vi "Create Ramp Array.vi"(0 "Start":dbl, 5 "Stop":dbl=1.0, 7 "Step":dbl, 11 "Error In":errorcluster) -> (4 "Ramp Pattern":dbl[](array[numeric]), 15 "Error Out":errorcluster)   [LabVIEW 2013]
uses:
  <vilib>/Analysis/1siggen.llb/Ramp Pattern by Delta.vi
  <vilib>/Analysis/NI_AALBase.lvlib
panel:
  out "samples":i32
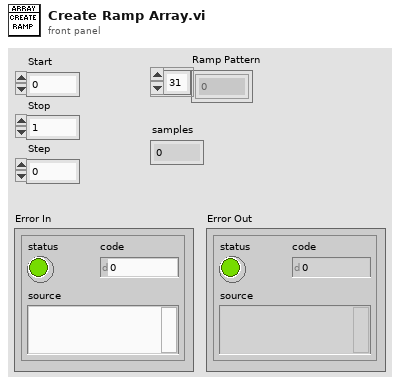
[diagram p1: front panel]
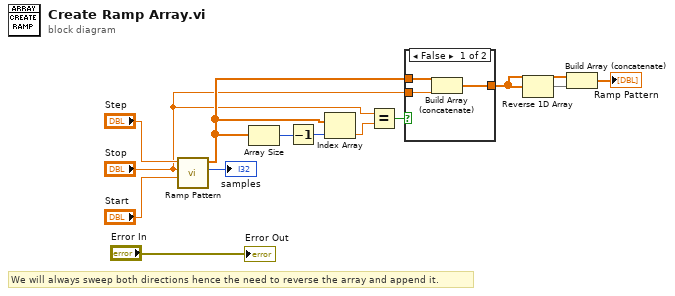
[diagram p0: block diagram]
diagram:
  # "We will always sweep both directions hence the need to reverse the array and append it."
  n1 = call-poly <vilib>:"Ramp Pattern.vi"("start"="Start", "end"="Stop", "delta"="Step") -> ("samples"=→"samples":i32, "Ramp Pattern"=w5:dbl[])  [unwired: 6 in, 1 out]
  n2 = Array Size(array=w5) -> (size(s)=w2:i32)
  n3 = Decrement(x=w2) -> (x-1=w1:i32)
  n4 = Index Array(array=w5, index=w1) -> (element=w7:dbl)
  n5 = Equal?(x="Stop", y=w7) -> (x = y?=w6:bool)
  n6 = case shown="False" w6 {
    tunnel: w5 -> [w16 w17]
    tunnel: [w14 w17] -> w4
    tunnel: "Stop" -> [w15 _]
    frame False {
      n7 = Build Array (concatenate)(w16, w15) -> (w14:dbl[])
    }
    frame True {
    }
  }
  n8 = Reverse 1D Array(array=w4) -> (reversed array=w10:dbl[])
  n9 = Build Array (concatenate)(w4, w10) -> (→"Ramp Pattern":dbl[])
  "Error Out" <- "Error In"
